vi "ST Locate.vi"(0 "VISA resource name":refnum<visa-resource-name>, 1 "error in (no error)":errorcluster) -> (2 "Result Code":i32, 3 "Ready and OK":bool, 4 "VISA resource name out":refnum<visa-resource-name>, 5 "Steps":i32[](array[numeric]), 6 "Angle":dbl[](array[numeric]), 7 "error out":errorcluster)   [LabVIEW 2009]
doc: "This VI get the location of the robot and presents the data in two array: motor steps and angle in radians.\nThe order of the data is :\nWAIST\nSHOULDER\nELBOW\nHAND\nWRIST"
panel:
  out "String Received":string
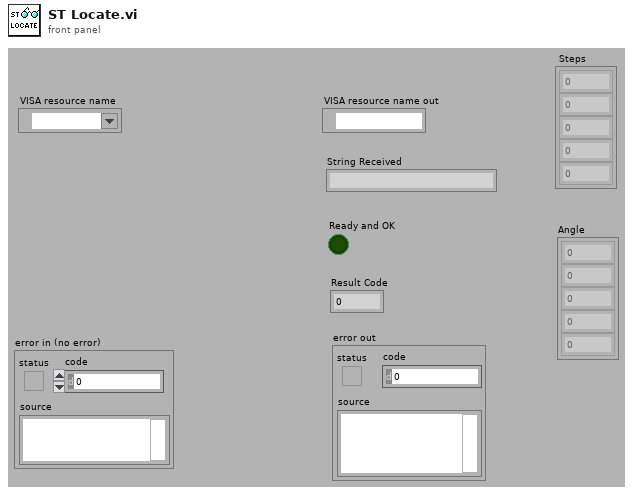
[diagram p1: front panel]
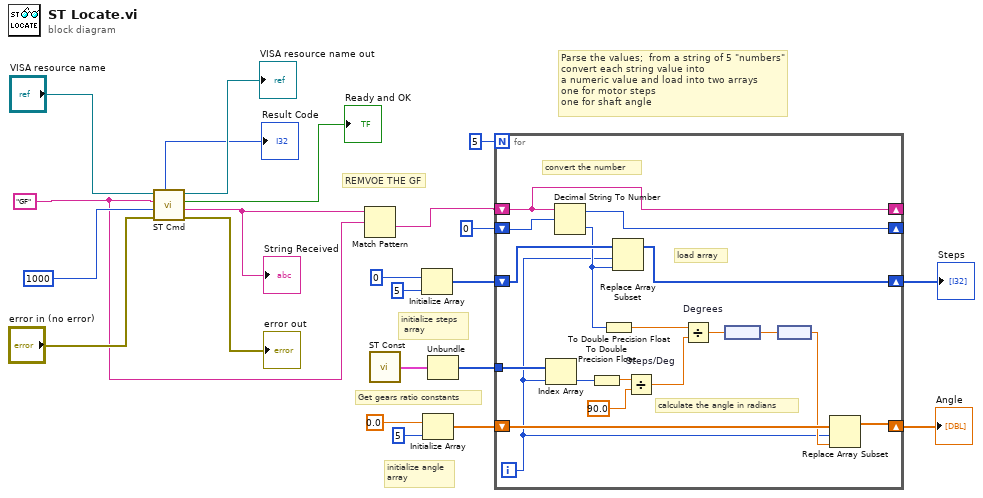
[diagram p0: block diagram]
diagram:
  w2 = "GF" ("Command String")
  # "REMVOE THE GF"
  # "Get gears ratio constants"
  # "initialize angle\narray"
  # "initialize steps\n array"
  # "Parse the values;  from a string of 5 \"numbers\"\nconvert each string value into \na numeric value and load into two arrays\none for motor steps\none for shaft angle"
  n1 = call "ST Cmd.vi"("error in (no error)"="error in (no error)", "Time Out"=1000, "Command String"=w2, "VISA resource name"="VISA resource name") -> ("error out"=→"error out":errorcluster, "String Received"=w3:string, "Ready and OK"=→"Ready and OK":bool, "VISA resource name out"=→"VISA resource name out":refnum<visa-resource-name>, "Result Code"=→"Result Code":i32)
  "String Received" <- w3
  n2 = Match Pattern(string=w3, regular expression=w2) -> (after substring=w1:string)  [unwired: 1 in, 3 out]
  n3 = call "ST Const.vi"() -> ("Robot Constants"=w10:cluster{i32[], i32[], dbl[]})
  n4 = Initialize Array(0 ("element"), 5 ("dimension size")) -> (w19:i32[])
  n5 = Initialize Array(0.0 ("element"), 5 ("dimension size")) -> (w6:dbl[])
  n6 = Unbundle(w10) -> (w9:i32[])  [unwired: 2 out]
  n7 = for {
    N: 5 -> [_]
    shift-right: [w38] -> _
    shift-left: w1 -> [w38]
    shift-right: [w37] -> _
    shift-left: 0 ("offset past token") -> [w36]
    shift-right: [w39] -> w18
    shift-left: w19 -> [w40]
    tunnel: w9 -> [w35]
    shift-right: [w23] -> w5
    shift-left: w6 -> [w26]
    i -> [w24]
    # "calculate the angle in radians"
    # "load array"
    # "convert the number"
    n8 = Index Array(array=w35, index=w24) -> (element=w32:i32)
    n9 = Decimal String To Number(string=w38, offset=w36) -> (offset past number=w37:i32, number=w30:i32)  [unwired: 1 in]
    n10 = To Double Precision Float(number=w32) -> (double precision float=w33:dbl)
    n11 = To Double Precision Float(number=w30) -> (double precision float=w29:dbl)
    n12 = Replace Array Subset(array=w40, new element=w30, index=w24) -> (w39:i32[])
    n13 = Divide "Steps/Deg"(x=w33, y=90.0) -> (x/y=w31:dbl)
    n14 = Divide "Degrees"(x=w29, y=w31) -> (x/y=w27:dbl)
    n15 = node(w27) -> (w28:dbl[unit])
    n16 = node(w28) -> (w25:dbl)
    n17 = Replace Array Subset(array=w26, new element=w25, index=w24) -> (w23:dbl[])
  }
  "Steps" <- w18
  "Angle" <- w5
